vi "AT Close A.vi"(8 "error in (no error)":errorcluster, 11 "Handle":i32) -> (0 "error out":errorcluster, 3 "Status":i32)   [LabVIEW 2019]
doc: "Close\n\nOutput:\n I32 Status\n\nInput:\n I32 Handle\n\nThis function is used to close a previously opened handle to a camera. The Handle parameter is the handle that was returned from the AT_Open function. The function should be called when you no longer wish to access the camera from your application usually at shutdown."
uses:
  atcoreA.dll
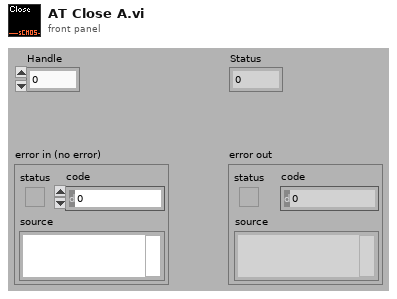
[diagram p1: front panel]
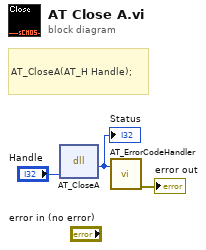
[diagram p0: block diagram]
diagram:
  # "AT_CloseA(AT_H Handle);"
  n1 = dll-call lib="atcoreA.dll" fn="AT_CloseA"("Handle"="Handle") -> ("Status"=w1:i32)  [unwired: 4 in, 2 out]
  "Status" <- w1
  n2 = call "AT_ErrorCodeHandler.vi"("Error"=w1) -> ("error out"=→"error out":errorcluster)  [unwired: 6 in]
